vi "AssertSubpanelVIExecNotBad.vi"(0 "VI Reference In":refnum<vi>, 1 "Test Label":string, 2 "delimiter (>>)":string=">>", 3 "Assert Only? (F)":bool, 5 "Control Path":string, 11 "Error In":errorcluster, 12 "Assert Interval(10 ms)":u32=10, 13 "Timeout(5 sec)":dbl=5.0) -> (4 "VI Reference Out":refnum<vi>, 6 "Test SubpanelVI Exec.State":T1(ring), 15 "Error Out":errorcluster)   [LabVIEW 2016, in "Drona.lvlib" / "AssertSubpanel.lvlib"]
doc: "Asserts if the Inserted VI in Subpanel is Not in Bad execution state.\nThe input control name is given as a string , incase of path, use delimiters inbetween the path."
uses:
  AssertSubpanel.lvlib
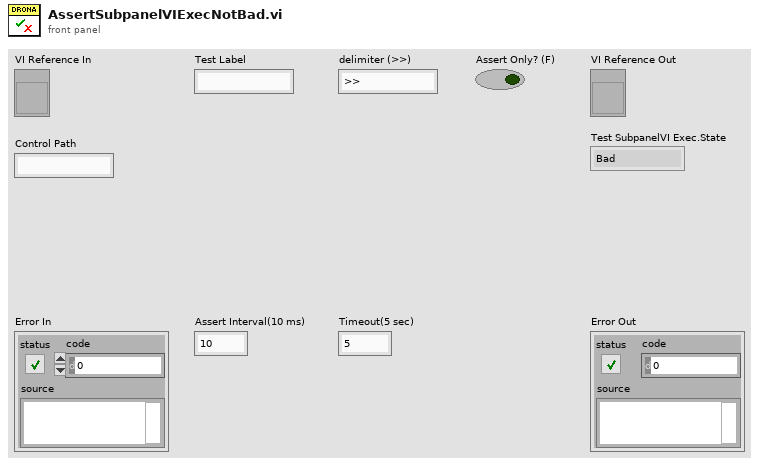
[diagram p1: front panel]
types:
  T1 = enum32{"Bad", "Idle", "Run top level", "Running"}
  T2 = enum32{"Bad", "Idle", "Run top level", "Running"}[]
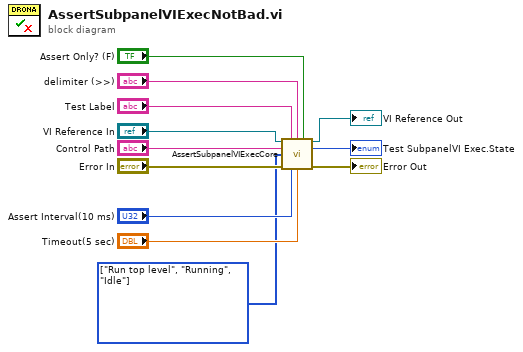
[diagram p0: block diagram]
diagram:
  w2 = T2 [enum."Run top level", enum."Running", enum."Idle"] items=["Bad", "Idle", "Run top level", "Running"] ("Execution:State")
  n1 = call "AssertSubpanelVIExecCore.vi"("VI Reference In"="VI Reference In", "Label"="Test Label", "delimiter (>>)"="delimiter (>>)", "Assert Only? (F)"="Assert Only? (F)", "Control Path"="Control Path", "Execution:State"=w2, "Error In"="Error In", "Assert Interval(10 ms)"="Assert Interval(10 ms)", "Timeout(5 sec)"="Timeout(5 sec)") -> ("VI Reference Out"=→"VI Reference Out":refnum<vi>, "Test SubpanelVI Exec.State"=→"Test SubpanelVI Exec.State":T1, "Error Out"=→"Error Out":errorcluster)  [unwired: 4 in]
